vi "euclidSpaceShift.vi"(4 "Y Vector Initialized Array":dbl[][](array[numeric]), 5 "Y Vector Component":dbl, 6 "X Vector Initialized Array":dbl[][](array[numeric]), 7 "X Vector Component":dbl, 8 "YMin":dbl, 9 "XMin":dbl, 10 "Y(i)":dbl, 11 "X(i)":dbl) -> (2 "Y Vector Component Array":dbl[][](array[numeric]), 3 "X Vector Component Array":dbl[][](array[numeric]))   [LabVIEW 2015]
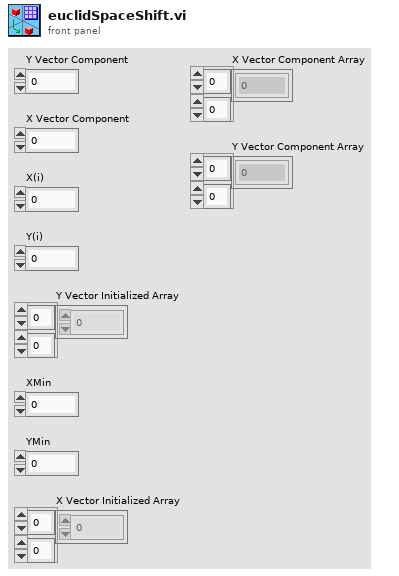
[diagram p1: front panel]
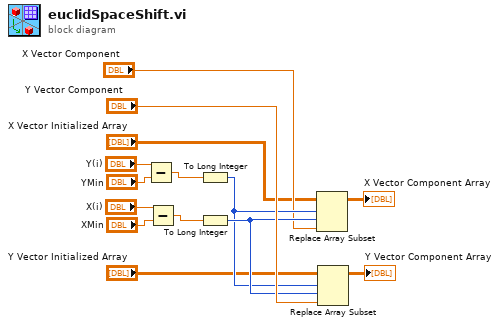
[diagram p0: block diagram]
diagram:
  n1 = Subtract(x="Y(i)", y="YMin") -> (x-y=w3:dbl)
  n2 = Subtract(x="X(i)", y="XMin") -> (x-y=w1:dbl)
  n3 = To Long Integer(number=w3) -> (32bit integer=w11:i32)
  n4 = To Long Integer(number=w1) -> (32bit integer=w12:i32)
  n5 = Replace Array Subset(array="X Vector Initialized Array", new element="X Vector Component", index (row)=w11, index (col)=w12) -> (→"X Vector Component Array":dbl[][])
  n6 = Replace Array Subset(array="Y Vector Initialized Array", new element="Y Vector Component", index (row)=w11, index (col)=w12) -> (→"Y Vector Component Array":dbl[][])
